vi "svx_Polar_SC_Menu.vi"(6 "Run Mode?":bool, 7 "State":T2={"Property Name"=[], "Container bounds"={"Width"=550, "Height"=250}, "Scale range"={"Maximum"=1.0, "Increment"=1.0}, "PointIdx"=0, "Marker list"=[], "Color settings"={"Arrow color"=16860, "Magnitude major grid"=13816530, "Magnitude minor grid"=16777216, "Phase grid"=13816530, "Phase scale marker text"=0}, "Magnitude scale name"="Magnitude", "Magnitude scale format string"="%#.2e", "MagnitudeScale:Visible"=TRUE, "MagnitudeScaleLabel:Visible"=TRUE, "PhaseScale:Visible"=TRUE, "Marker:Visible"=TRUE, "Cursor:Visible"=FALSE, "CursorName:Visible"=TRUE, "Autoscale"=TRUE, "Marker color"=16860, "Line color"=16711680, "Cursor color"=16711680, "Magnitude scale marker color"=0, "Plot.Line Style"=0, "Plot.Line Width"=0, "Plot.Point Style"=0, "Cursor.Line Style"=0, "Cursor.Line Width"=0, "Cursor.Point Style"=0, "Cursor.Style"=4, "Marker.Point Style"=2, "Point/fill color"=16711680, "Background color"=16777225, "Cursor name"="", "Cursor Release"=refnum, "Scale Range Change"=refnum, "data size(s)"=[], "Selectors:Visible"=TRUE, "Selector:ring Strings"={"Selector:Custom Strings"=FALSE, "Selector:Row Strings []"=[], "Selector:Column Strings []"=[], "User:Row Strings []"=[], "User:Column Strings []"=[]}, "Lock Cursor Info Position"=FALSE, "CursLoc"={"magnitude"=0.0, "phase"=0.0, "time/rev/RPM"=0.0}, "Plot Area:Position"={"Left"=0, "Top"=0}, "Plot Area:Size"={"Width"=0, "Height"=0}, "Marker.Style"=0, "Indication Arcs"=[], "Arc.Selector"=0, "customized marker"=[], "tree Width"=0, " Parents Tags"=[], "Children Tags"=[], "open?"=[], "index"=[{"row index"=0, "column index"=0}], "Label"="", "custom strings changed"=FALSE, "Owning VI"=refnum, "Legend BG color"=16777225, "Legend font color"=0, "column Width"=203, "attribute"=variant}, 10 "Refnum":refnum<vi>, 11 "MenuRef":refnum<k9>) -> ()   [LabVIEW 2017, in "SVX Polar Plot.xctl"]
uses:
  <vilib>/addons/_XControls/Polar Plot/SVX Polar Plot.xctl
  <vilib>/addons/_XControls/Polar Plot/subVIs/svx_Polar_Plot_Internal_State.ctl
  <vilib>/addons/_XControls/Polar Plot/subVIs/svx_Polar_Indication_Arcs.ctl
  <vilib>/addons/_XControls/Polar Plot/subVIs/svx_Polar_Customized_Markers.ctl
panel:
  in  "run-time menu":T1(array[cluster])=[{"menu tag"="", "items to delete"=["APP_SC_VISIBLE_ITEMS", "APP_SC_VISIBLE_ITEMS", "APP_SC_AUTOSCALE_X", "APP_SC_AUTOSCALE_Y", "APP_SC_SMOOTH_UPDATES", "APP_SC_PROPERTIES", "APP_SC_SHOW_DIAGRAM", "APP_SC_CREATE_ANNOTATION", "APP_SC_DELETE_ALL_ANNOTATIONS", "APP_SC_CLEAR_GRAPH"], "new menu"=[{"item names"="Visible Items", "item tags"="USER_SC_VISIBLE_ITEMS", "after item"=""}, {"item names"="Clear Graph", "item tags"="USER_SC_CLEAR_GRAPH", "after item"="USER_SC_VISIBLE_ITEMS"}, {"item names"="Autoscale", "item tags"="USER_SC_AUTOSCALE", "after item"="APP_SEPERATOR"}, {"item names"="-", "item tags"="APP_SC_SEPARATOR_2", "after item"="USER_SC_AUTOSCALE"}, {"item names"="Acceptance Region", "item tags"="USER_SC_ACCEPTANCE_REGION", "after item"="APP_SC_SEPARATOR_2"}], "root?"=TRUE}, {"menu tag"="USER_SC_VISIBLE_ITEMS", "items to delete"=["APP_SC_PLOT_LEGEND", "APP_SC_SCALE_LEGEND", "APP_SC_CURSOR_LEGEND", "APP_SC_X_SCROLLBAR", "APP_SC_X_SCALE", "APP_SC_Y_SCALE", "APP_SC_UNIT_LABEL"], "new menu"=[{"item names"="Plot Legend", "item tags"="USER_SC_PLOT_LEGEND", "after item"="APP_SC_SEPERATOR"}, {"item names"="-", "item tags"="APP_SC_SEPERATOR2", "after item"="USER_SC_PLOT_LEGEND"}, {"item names"="Magnitude Scale", "item tags"="USER_SC_MAGNITUDE_SCALE", "after item"="APP_SC_SEPERATOR2"}, {"item names"="Phase Scale", "item tags"="USER_SC_PHASE_SCALE", "after item"="USER_SC_MAGNITUDE_SCALE"}, {"item names"="-", "item tags"="APP_SC_SEPERATOR3", "after item"="USER_SC_PHASE_SCALE"}, {"item names"="Cursor", "item tags"="USER_SC_CURSOR", "after item"="APP_SC_SEPERATOR3"}, {"item names"="Cursor Info", "item tags"="USER_SC_CURSOR_INFO", "after item"="USER_SC_CURSOR"}, {"item names"="Lock Cursor Info Position", "item tags"="USER_SC_LOCK_CURSOR_INFO", "after item"="USER_SC_CURSOR_INFO"}, {"item names"="Marker", "item tags"="USER_SC_MARKER", "after item"="USER_SC_LOCK_CURSOR_INFO"}], "root?"=FALSE}]
  in  "edit-time menu":T1(array[cluster])=[{"menu tag"="", "items to delete"=["APP_SC_VISIBLE_ITEMS", "APP_SC_VISIBLE_ITEMS", "APP_SC_AUTOSCALE_X", "APP_SC_AUTOSCALE_Y", "APP_SC_SMOOTH_UPDATES", "APP_SC_PROPERTIES"], "new menu"=[{"item names"="Visible Items", "item tags"="USER_SC_VISIBLE_ITEMS", "after item"=""}, {"item names"="Autoscale", "item tags"="USER_SC_AUTOSCALE", "after item"="APP_SEPERATOR"}, {"item names"="-", "item tags"="APP_SC_SEPARATOR_4", "after item"="USER_SC_AUTOSCALE"}, {"item names"="Properties", "item tags"="USER_SC_PROPERTIES", "after item"="APP_SC_SEPARATOR_4"}], "root?"=TRUE}, {"menu tag"="USER_SC_VISIBLE_ITEMS", "items to delete"=["APP_SC_PLOT_LEGEND", "APP_SC_SCALE_LEGEND", "APP_SC_CURSOR_LEGEND", "APP_SC_X_SCROLLBAR", "APP_SC_X_SCALE", "APP_SC_Y_SCALE", "APP_SC_UNIT_LABEL"], "new menu"=[{"item names"="Label", "item tags"="USER_SC_LABEL", "after item"=""}, {"item names"="Caption", "item tags"="USER_SC_CAPTION", "after item"="USER_SC_LABEL"}, {"item names"="-", "item tags"="APP_SC_SEPERATOR", "after item"="USER_SC_CAPTION"}, {"item names"="Plot Legend", "item tags"="USER_SC_PLOT_LEGEND", "after item"="APP_SC_SEPERATOR"}, {"item names"="-", "item tags"="APP_SC_SEPERATOR2", "after item"="USER_SC_PLOT_LEGEND"}, {"item names"="Magnitude Scale", "item tags"="USER_SC_MAGNITUDE_SCALE", "after item"="APP_SC_SEPERATOR2"}, {"item names"="Phase Scale", "item tags"="USER_SC_PHASE_SCALE", "after item"="USER_SC_MAGNITUDE_SCALE"}, {"item names"="-", "item tags"="APP_SC_SEPERATOR3", "after item"="USER_SC_PHASE_SCALE"}, {"item names"="Cursor", "item tags"="USER_SC_CURSOR", "after item"="APP_SC_SEPERATOR3"}, {"item names"="Cursor Info", "item tags"="USER_SC_CURSOR_INFO", "after item"="USER_SC_CURSOR"}, {"item names"="Lock Cursor Info Position", "item tags"="USER_SC_LOCK_CURSOR_INFO", "after item"="USER_SC_CURSOR_INFO"}, {"item names"="Marker", "item tags"="USER_SC_MARKER", "after item"="USER_SC_LOCK_CURSOR_INFO"}], "root?"=FALSE}, {"menu tag"="APP_SC_ADVANCED", "items to delete"=["APP_SC_KEY_NAVIGATION", "APP_SC_CUSTOMIZE", "APP_SC_SHOW_DIAGRAM"], "new menu"=[], "root?"=FALSE}, {"menu tag"="APP_SC_DATA_OPERATIONS", "items to delete"=["APP_SC_CREATE_ANNOTATION", "APP_SC_DELETE_ALL_ANNOTATIONS", "APP_SC_CLEAR_GRAPH"], "new menu"=[{"item names"="Clear Graph", "item tags"="USER_SC_CLEAR_GRAPH", "after item"=""}], "root?"=FALSE}, {"menu tag"="APP_SC_Advanced", "items to delete"=["APP_SC_RUN-TIME_SC_MENU"], "new menu"=[], "root?"=FALSE}]
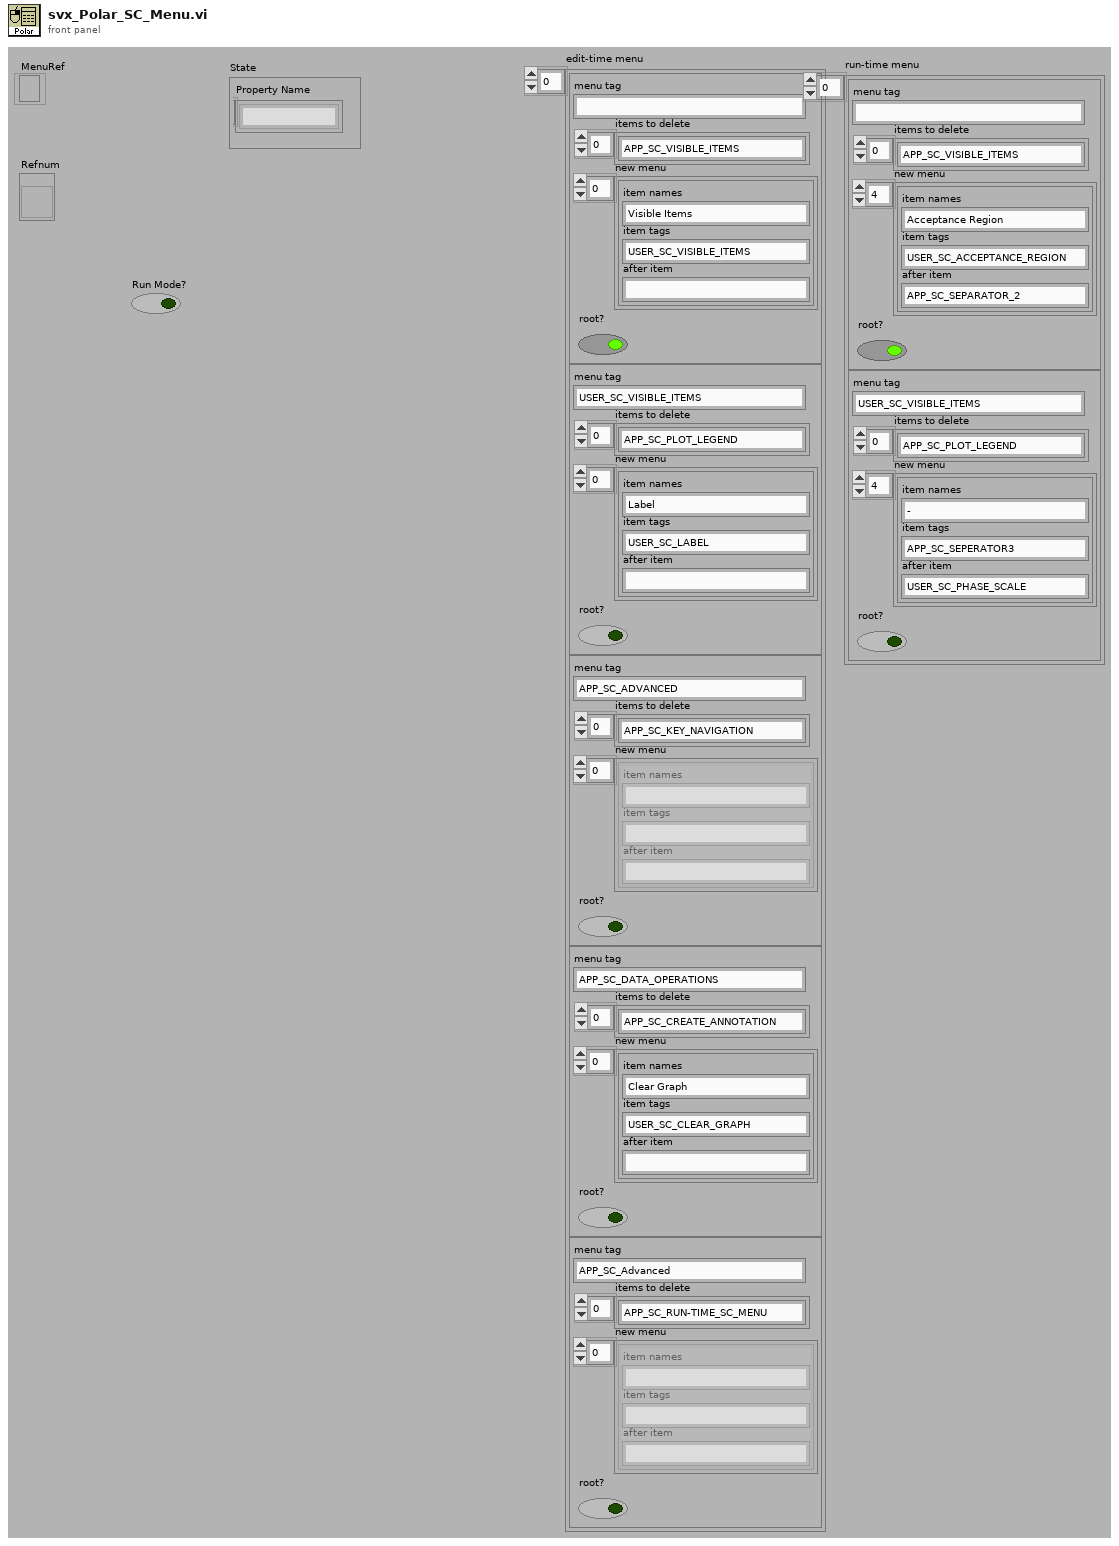
[diagram p1: front panel]
types:
  T1 = cluster{"menu tag":string, "items to delete":string[], "new menu":cluster{"item names":string, "item tags":string, "after item":string}[], "root?":bool}[]
  T2 = typedef "SVX Polar Plot.xctl/svx_Polar_Plot_Internal_State.ctl" = cluster{"Property Name":string[], "Container bounds":cluster{"Width":u32, "Height":u32}, "Scale range":cluster{"Maximum":dbl, "Increment":dbl}, "PointIdx":i32, "Marker list":cluster{"Name":string, "Color":u32, "Style":u8, "Point Style":u8, "Name Visible":bool, "Allow Drag":bool, "Annotation Mode":u32, "Plot":i32, "Index":i32, "Position":cluster{"X":dbl, "Y":dbl}, "X Scale":u32, "Y Scale":u32, "Show Arrow":bool, "Lock Name":bool, "Plot Area":i32, "Label Offset":cluster{"X":dbl, "Y":dbl}}[], "Color settings":cluster{"Arrow color":u32, "Magnitude major grid":u32, "Magnitude minor grid":u32, "Phase grid":u32, "Phase scale marker text":u32}, "Magnitude scale name":string, "Magnitude scale format string":string, "MagnitudeScale:Visible":bool, "MagnitudeScaleLabel:Visible":bool, "PhaseScale:Visible":bool, "Marker:Visible":bool, "Cursor:Visible":bool, "CursorName:Visible":bool, "Autoscale":bool, "Marker color":u32, "Line color":u32, "Cursor color":u32, "Magnitude scale marker color":u32, "Plot.Line Style":i32, "Plot.Line Width":i32, "Plot.Point Style":i32, "Cursor.Line Style":i32, "Cursor.Line Width":i32, "Cursor.Point Style":i32, "Cursor.Style":i32, "Marker.Point Style":i32, "Point/fill color":u32, "Background color":u32, "Cursor name":string, "Cursor Release":refnum<user-event>, "Scale Range Change":refnum<user-event>, "data size(s)":i32[], "Selectors:Visible":bool, "Selector:ring Strings":cluster{"Selector:Custom Strings":bool, "Selector:Row Strings []":string[], "Selector:Column Strings []":string[], "User:Row Strings []":string[], "User:Column Strings []":string[]}, "Lock Cursor Info Position":bool, "CursLoc":cluster{"magnitude":dbl, "phase":dbl, "time/rev/RPM":dbl}, "Plot Area:Position":cluster{"Left":i32, "Top":i32}, "Plot Area:Size":cluster{"Width":u32, "Height":u32}, "Marker.Style":i32, "Indication Arcs":T3, "Arc.Selector":u16, "customized marker":T4, "tree Width":u32, " Parents Tags":string[], "Children Tags":string[], "open?":bool[], "index":cluster{"row index":i32, "column index":i32}[], "Label":string, "custom strings changed":bool, "Owning VI":refnum<vi>, "Legend BG color":u32, "Legend font color":u32, "column Width":u32, "attribute":variant}
  T3 = typedef "SVX Polar Plot.xctl/svx_Polar_Indication_Arcs.ctl" = cluster{"Name":string, "Start radius":dbl, "End radius":dbl, "Line Style":i32, "Line Width":i32, "Border color":u32, "Fill color":u32, "Start angle":i16, "End angle":i16, "Visible":bool}[]
  T4 = typedef "SVX Polar Plot.xctl/svx_Polar_Customized_Markers.ctl" = cluster{"Name":string, "Color":u32, "Style":u8, "Point Style":u8, "Name Visible":bool, "Allow Drag":bool, "Annotation Mode":u32, "Plot":i32, "Index":i32, "Position":cluster{"Magnitude":dbl, "Phase":dbl}, "X Scale":u32, "Y Scale":u32, "Show Arrow":bool, "Lock Name":bool, "Plot Area":i32, "Label Offset":cluster{"Magnitude":dbl, "Phase":dbl}}[]
  T5 = cluster{"item names":string, "item tags":string, "after item":string}[]
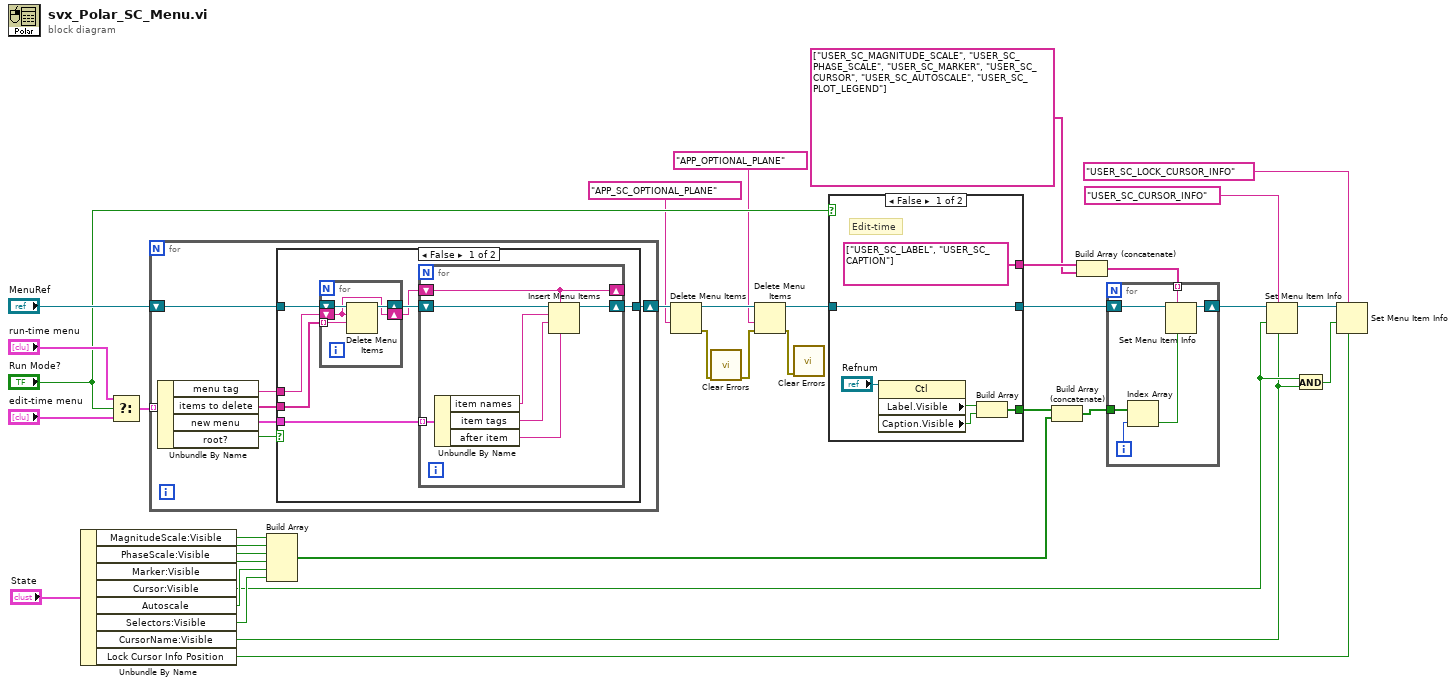
[diagram p0: block diagram]
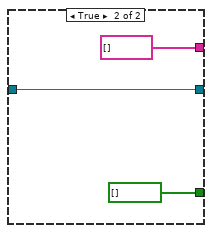
[diagram p2: hidden frame]
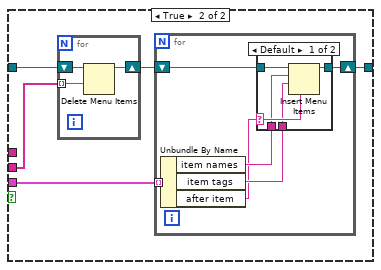
[diagram p3: hidden frame]
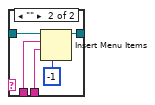
[diagram p4: hidden frame]
diagram:
  n1 = Unbundle By Name("State") -> ("MagnitudeScale:Visible"=w26:bool, "PhaseScale:Visible"=w25:bool, "Marker:Visible"=w24:bool, "Cursor:Visible"=w3:bool, "Autoscale"=w23:bool, "Selectors:Visible"=w16:bool, "CursorName:Visible"=w2:bool, "Lock Cursor Info Position"=w4:bool)
  n2 = Select(t="run-time menu", s="Run Mode?", f="edit-time menu") -> (s? t:f=w31:T1)
  n3 = for {
    tunnel: w31 -> [w41] mode=indexing
    shift-right: [w36] -> w33
    shift-left: "MenuRef" -> [w40]
    n4 = Unbundle By Name(w41) -> ("menu tag"=w39:string, "items to delete"=w38:string[], "new menu"=w37:T5, "root?"=w35:bool)
    n5 = case shown="False" w35 {
      tunnel: w40 -> [w48 w64]
      tunnel: w39 -> [w47 _]
      tunnel: w38 -> [w46 w63]
      tunnel: w37 -> [w43 w61]
      tunnel: [w42 w60] -> w36
      frame False {
        n6 = for {
          shift-right: [w58] -> w45
          shift-left: w48 -> [w59]
          shift-right: [w56] -> w44
          shift-left: w47 -> [w56]
          tunnel: w46 -> [w57] mode=indexing
          n7 = Delete Menu Items(7:w57, 8:w56, 9:w59) -> (3:w58:refnum<k9>)  [unwired: 1 in, 1 out]
        }
        n8 = for {
          shift-right: [w49] -> w42
          shift-left: w45 -> [w55]
          shift-right: [w54] -> _
          shift-left: w44 -> [w54]
          tunnel: w43 -> [w53] mode=indexing
          n9 = Unbundle By Name(w53) -> ("item names"=w52:string, "item tags"=w51:string, "after item"=w50:string)
          n10 = Insert Menu Items(4:w50, 5:w54, 7:w51, 8:w52, 9:w55) -> (3:w49:refnum<k9>)  [unwired: 1 in, 2 out]
        }
      }
      frame True {
        n11 = for {
          shift-right: [w82] -> w62
          shift-left: w64 -> [w83]
          tunnel: w63 -> [w81] mode=indexing
          n12 = Delete Menu Items(7:w81, 9:w83) -> (3:w82:refnum<k9>)  [unwired: 2 in, 1 out]
        }
        n13 = for {
          shift-right: [w70] -> w60
          shift-left: w62 -> [w69]
          tunnel: w61 -> [w68] mode=indexing
          n14 = Unbundle By Name(w68) -> ("item names"=w67:string, "item tags"=w66:string, "after item"=w65:string)
          n15 = case shown="Default" w65 {
            selector: w65 -> [w73 _]
            tunnel: [w74 w80] -> w70
            tunnel: w69 -> [w75 w79]
            tunnel: w67 -> [w72 w78]
            tunnel: w66 -> [w71 w77]
            frame Default {
              n16 = Insert Menu Items(4:w73, 7:w71, 8:w72, 9:w75) -> (3:w74:refnum<k9>)  [unwired: 2 in, 2 out]
            }
            frame "" {
              n17 = Insert Menu Items(4:-1, 7:w77, 8:w78, 9:w79) -> (3:w80:refnum<k9>)  [unwired: 2 in, 2 out]
            }
          }
        }
      }
    }
  }
  n18 = Build Array(w26, w25, w24, w3, w23, w16) -> (w18:bool[])
  n19 = Delete Menu Items(7:"APP_SC_OPTIONAL_PLANE" ("menu tag"), 9:w33) -> (0:w10:errorcluster, 3:w14:refnum<k9>)  [unwired: 2 in]
  n20 = call <vilib>:"Clear Errors.vi"("error in (no error)"=w10) -> ("error out"=w9:errorcluster)  [unwired: 5 in, 1 out]
  n21 = Delete Menu Items(6:w9, 7:"APP_OPTIONAL_PLANE" ("menu tag"), 9:w14) -> (0:w8:errorcluster, 3:w13:refnum<k9>)  [unwired: 1 in]
  n22 = call <vilib>:"Clear Errors.vi"("error in (no error)"=w8) -> ()  [unwired: 5 in, 2 out]
  n23 = case shown="False" "Run Mode?" {
    tunnel: w13 -> [w84 w91]
    tunnel: [string[] ["USER_SC_LABEL", "USER_SC_CAPTION"] string[] []] -> w22
    tunnel: [w85 bool[] []] -> w19
    tunnel: [w84 w91] -> w28
    frame False {
      # "Edit-time"
      n24 = property class="Ctl"(reference="Refnum") -> ("Label.Visible"=w88:bool, "Caption.Visible"=w87:bool)  [unwired: 1 in, 2 out]
      n25 = Build Array(w88, w87) -> (w85:bool[])
    }
    frame True {
    }
  }
  n26 = Build Array (concatenate)(w19, w18) -> (w17:bool[])
  n27 = Build Array (concatenate)(w22, string[] ["USER_SC_MAGNITUDE_SCALE", "USER_SC_PHASE_SCALE", "USER_SC_MARKER", "USER_SC_CURSOR", "USER_SC_AUTOSCALE", "USER_SC_PLOT_LEGEND"]) -> (w20:string[])
  n28 = for {
    shift-right: [w97] -> w15
    shift-left: w28 -> [w98]
    tunnel: w20 -> [w96] mode=indexing
    tunnel: w17 -> [w94]
    i -> [w95]
    n29 = Index Array(array=w94, index=w95) -> (element=w93:bool)
    n30 = Set Menu Item Info(6:w93, 7:w96, 11:w98) -> (3:w97:refnum<k9>)  [unwired: 4 in, 1 out]
  }
  n31 = Set Menu Item Info(6:w2, 7:"USER_SC_CURSOR_INFO", 9:w3, 11:w15) -> (3:w6:refnum<k9>)  [unwired: 3 in, 1 out]
  n32 = And(x=w3, y=w2) -> (x .and. y?=w1:bool)
  n33 = Set Menu Item Info(6:w4, 7:"USER_SC_LOCK_CURSOR_INFO", 9:w1, 11:w6) -> ()  [unwired: 3 in, 2 out]
